vi "QuP Multiplexer Control.vi"(11 "Do full quit? (T)":bool=TRUE) -> ()   [LabVIEW 2020, in "QuPMXdriver.lvlib"]
uses:
  QuPMXdriver.lvlib
  91754cce-ab52-4237-b78a-64c01c446f44.vi
  32ad12f4-2c8c-4504-800a-0d774754ae80.vi
  bf4f7028-8ca7-4759-aadb-7144e2be3c91.vi
  040f1b57-66c1-4072-aa26-6ea72dd8171f.vi
  6aed5eb3-691d-4dc6-b830-00691c629857.vi
  Sequence Editor.vi
  <vilib>/Comparison/Equal/Equal Functor/Equal Functor.lvclass
panel:
  in  "Init-reset":bool caption="Reset after connect:"
  in  "Init-idquery":bool=TRUE caption="ID query after connect:"
  out "FPdisAcon":refnum<vi>[](array[refnum])
  in  "Startup delay (ms)":u32=2000
  in  "disconnect":bool
  out "dummy for event \"check channels\"":bool
  in  "Set to sequence line:":i32=2 min=1 step=1
  in  "set sq line":bool
  out "Connected\nboards":bool[](array[boolean])
  in  "Get sq from MX":bool
  in  "Load sq to MX":bool
  in  "no sequences get":bool
  out "Number of sequence lines:":i32 min=0 step=1
  in  "sequence editor":bool
  out "Guards ref array":refnum<vi>[][](array[refnum])
  in  "G5C1":bool
  in  "G5C2":bool
  in  "G6C1":bool
  in  "G6C2":bool
  in  "G4C1":bool
  in  "G4C2":bool
  in  "G3C1":bool
  in  "G3C2":bool
  in  "G2C1":bool
  in  "G2C2":bool
  in  "G1C1":bool
  in  "G1C2":bool
  out "No. of connected slave boards:":u32
  out "Slaves ref array":refnum<vi>[][](array[refnum])
  in  "S5C1":bool
  in  "S5C2":bool
  in  "S6C1":bool
  in  "S6C2":bool
  in  "S4C1":bool
  in  "S4C2":bool
  in  "S3C1":bool
  in  "S3C2":bool
  in  "S2C1":bool
  in  "S2C2":bool
  in  "S1C1":bool
  in  "S1C2":bool
  in  "connect":bool
  in  "Get Status":bool
  out "Ready?":bool=TRUE
  out "Enabled":bool=TRUE
  in  "check channels":bool
  in  "delay get":bool
  in  "delay set":bool
  in  "Enable\nDelay (ms)":dbl=2.0 min=0.8
  in  "timer get":bool
  in  "timer set":bool
  in  "Timer (ms)":i32=1000 min=0 step=1
  in  "Trigger polarity":enum32{"Positive", "Negative"}(radio)
  in  "Trigger source":enum32{"Internal", "External"}(radio)
  out "FPenAcon":refnum<vi>[](array[refnum])
  in  "Operation":enum32{"Remote", "Local"}(radio)=enum."Local"
  out "ID:":string
  in  "reset":bool
  in  "clear":bool
  in  "stop":bool
  in  "start":bool
  in  "resume":bool
  in  "pause":bool
  in  "Close":bool
  out "error":errorcluster
  in  "VISA":refnum<visa-resource-name>
  # "Connect"
  # "Status"
  # "Channels"
  # "Properties"
  # "Slave boards"
  # "1       2      3      4      5      6"
  # "Channel 1"
  # "Channel 2"
  # "1       2      3      4      5      6"
  # "Guards"
  # "Channel 1"
  # "These are buttons,\nclick it!"
  # "Channel 2"
  # "Sequence"
  # "Error"
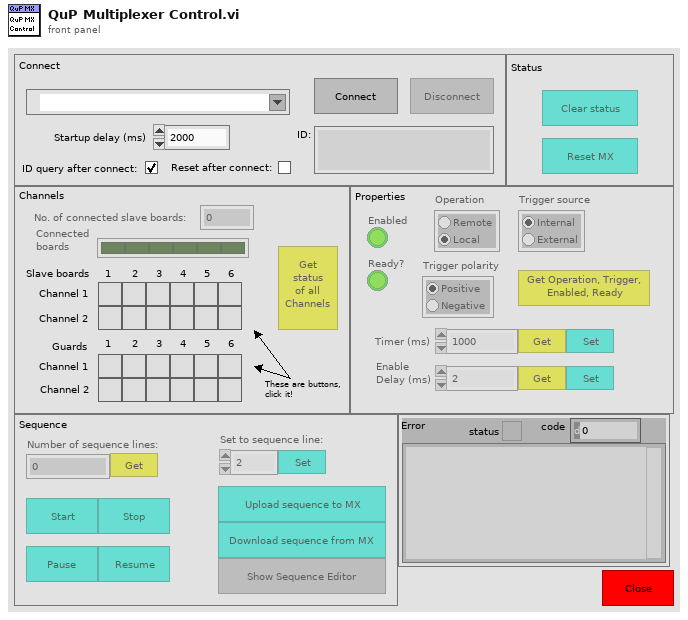
[diagram p1: front panel]
types:
  T1 = enum8{"Enabled", "Disabled", "Disabled and Grayed Out"}
  T2 = enum32{"Invalid", "Standard", "Closed", "Hidden", "Minimized", "Maximized"}
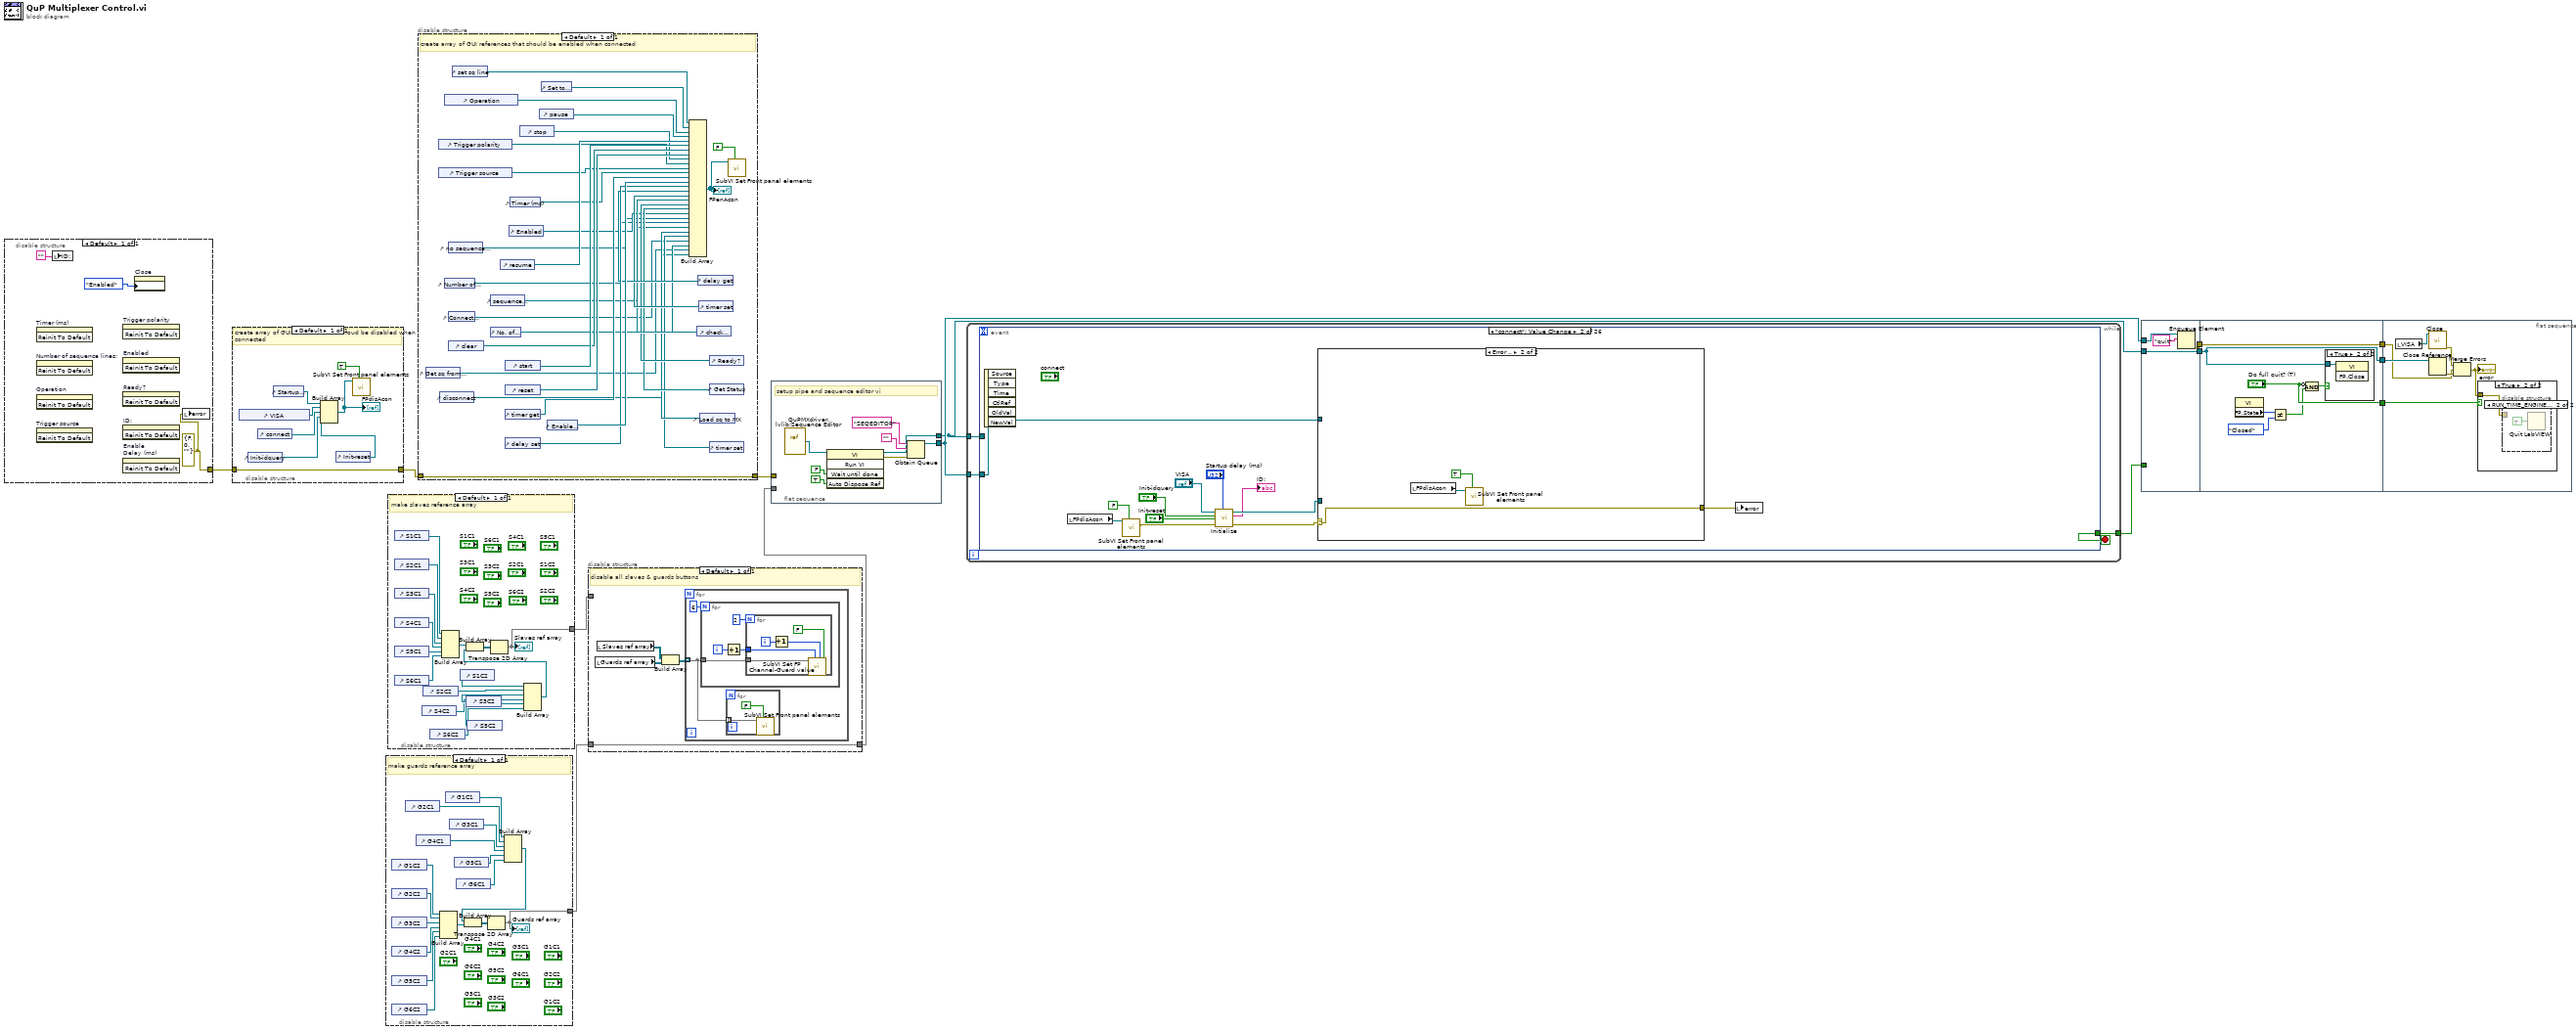
[diagram p0: block diagram]
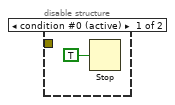
[diagram p4: hidden frame]
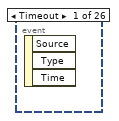
[diagram p5: hidden frame]
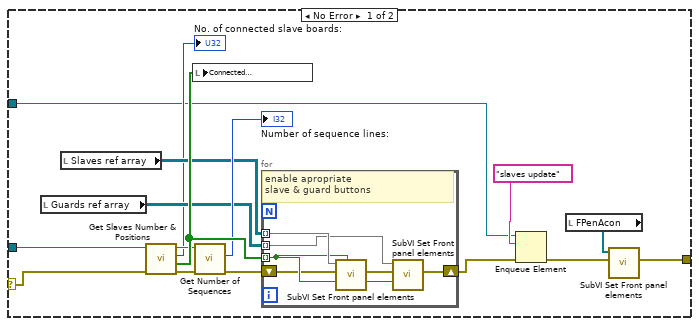
[diagram p6: hidden frame]
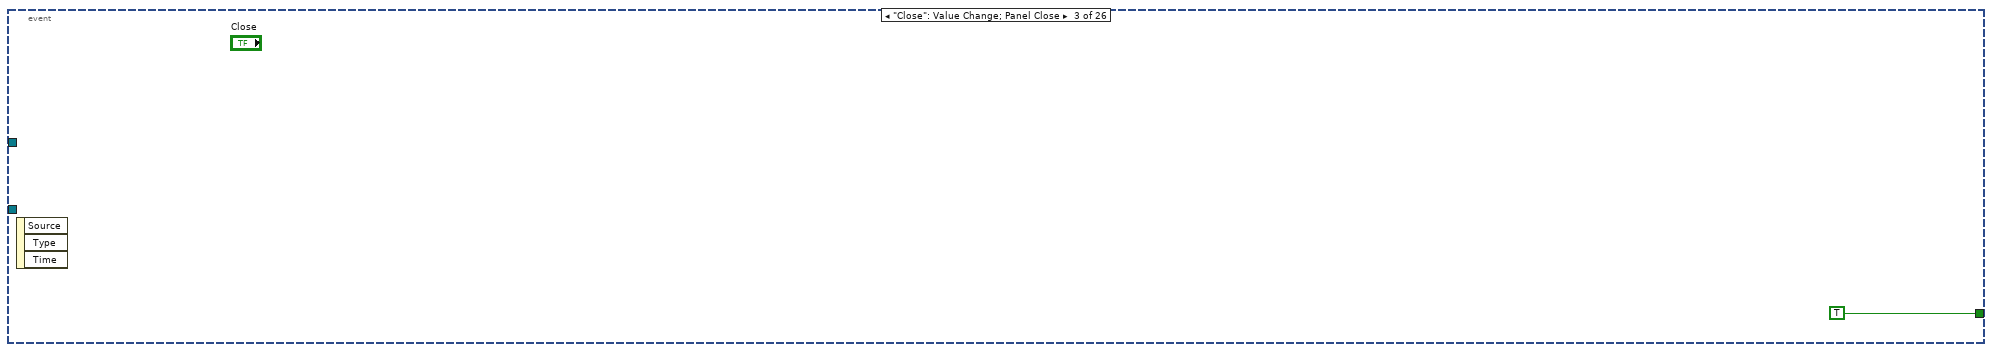
[diagram p7: hidden frame]
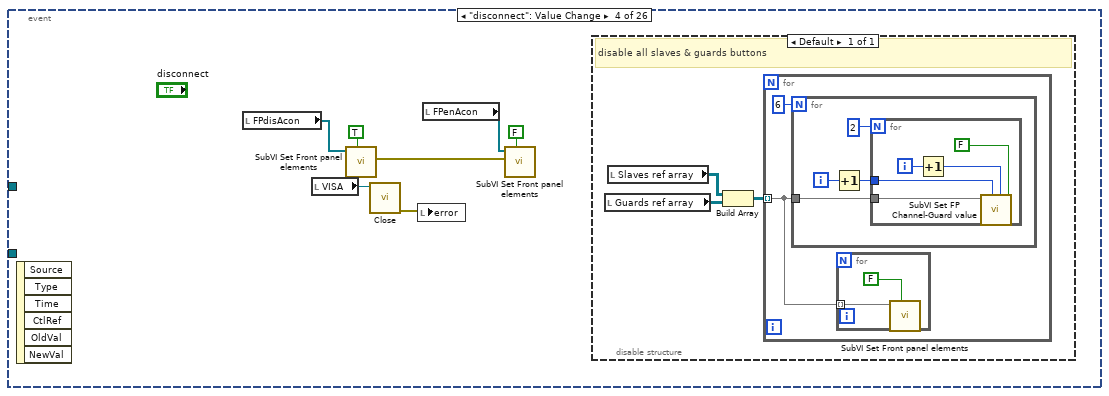
[diagram p8: hidden frame]
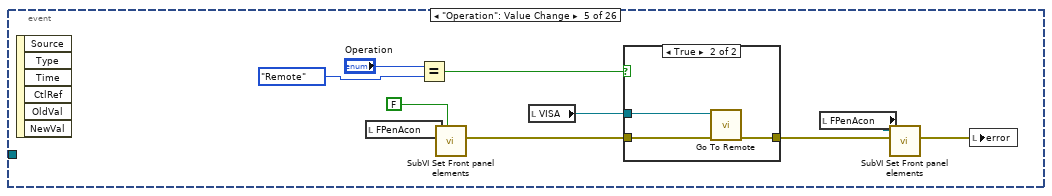
[diagram p9: hidden frame]
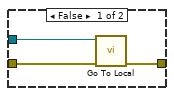
[diagram p10: hidden frame]
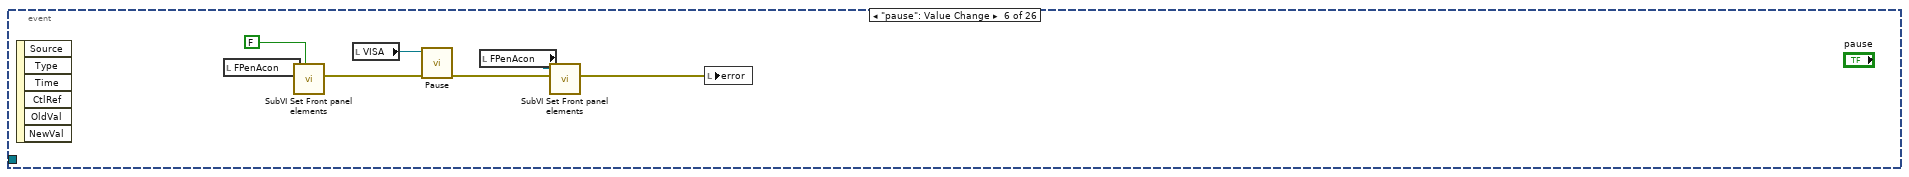
[diagram p11: hidden frame]
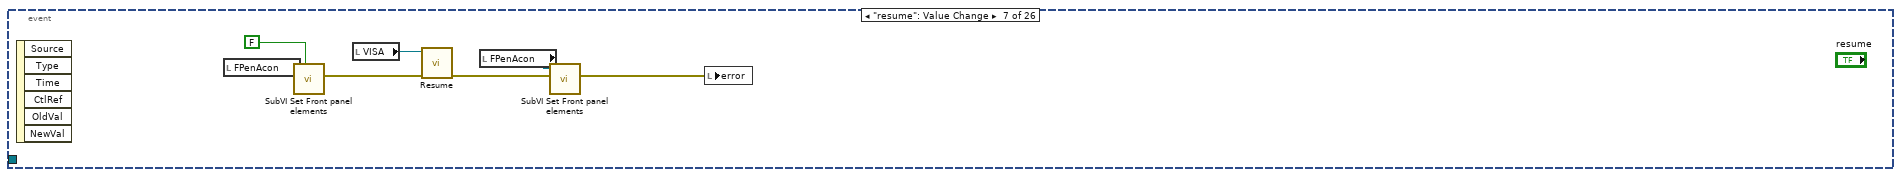
[diagram p12: hidden frame]
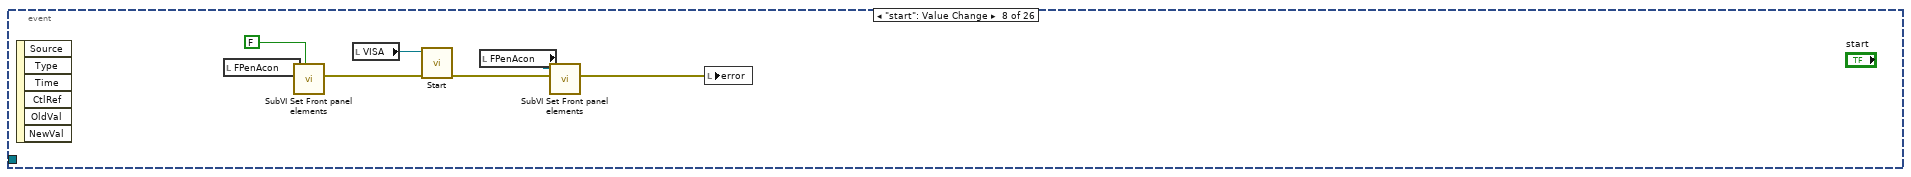
[diagram p13: hidden frame]
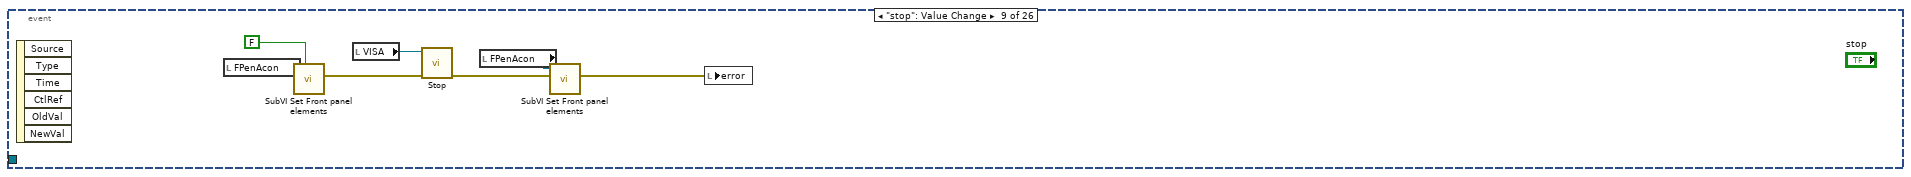
[diagram p14: hidden frame]
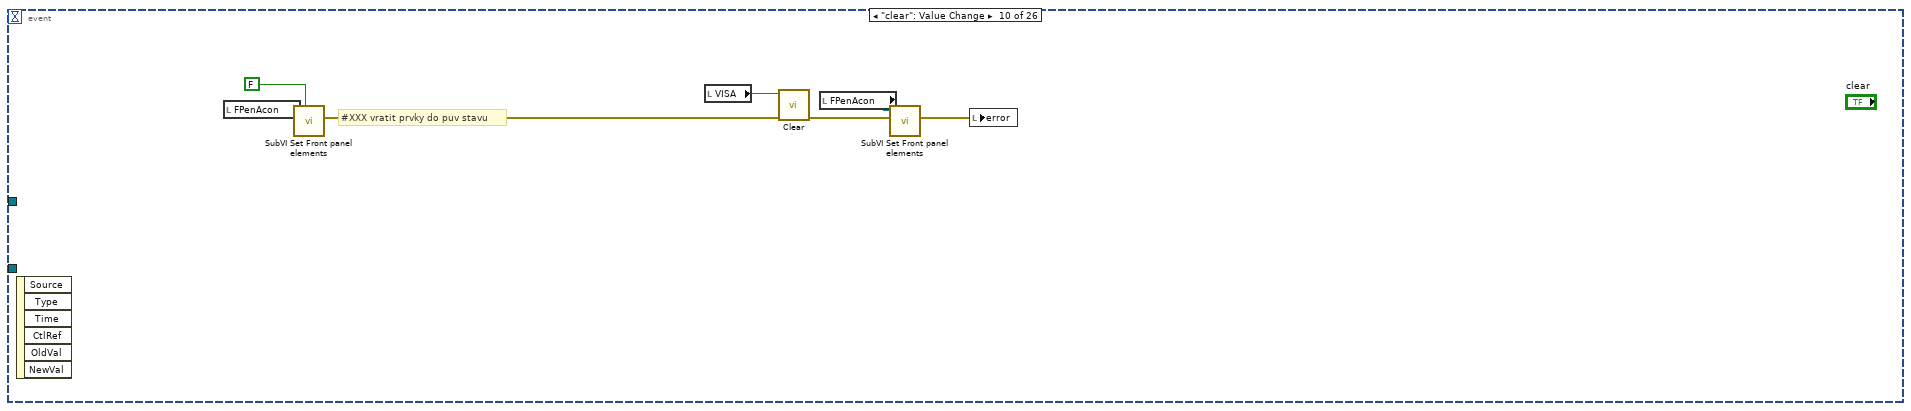
[diagram p15: hidden frame]
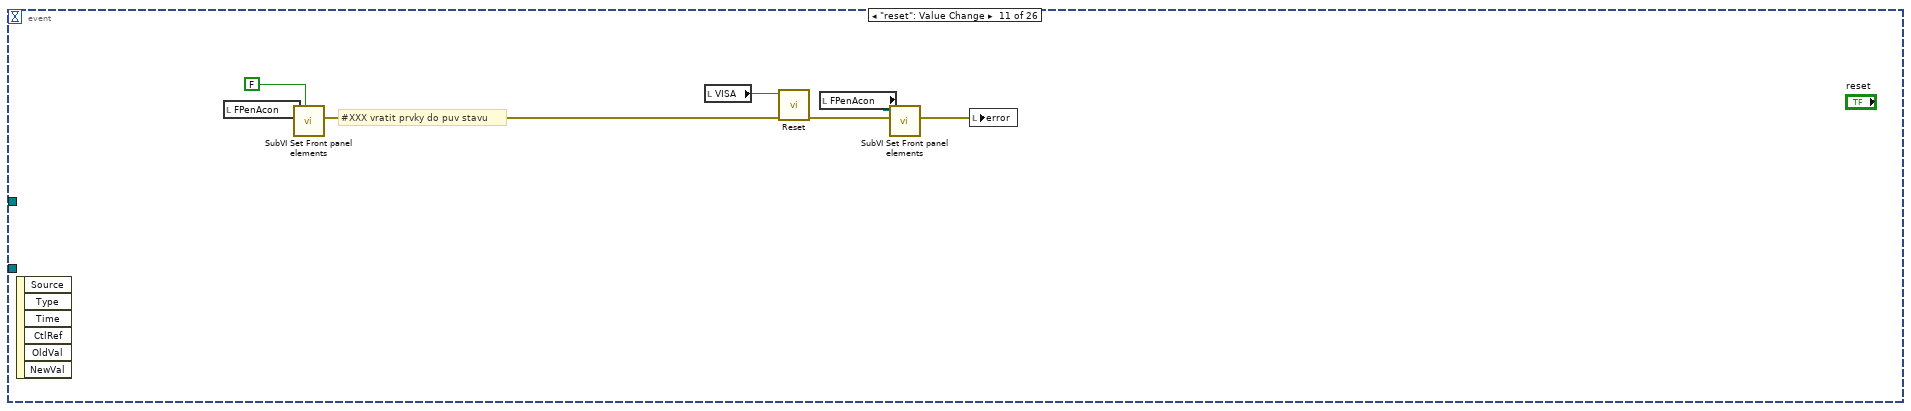
[diagram p16: hidden frame]
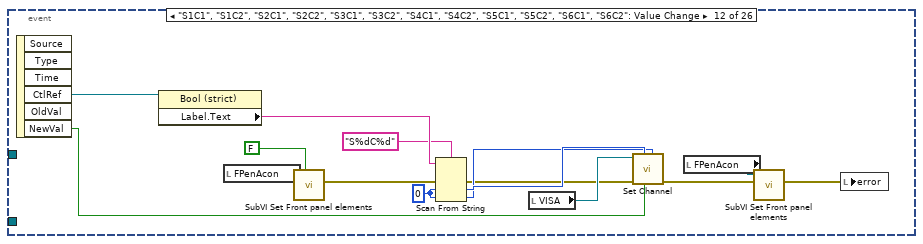
[diagram p17: hidden frame]
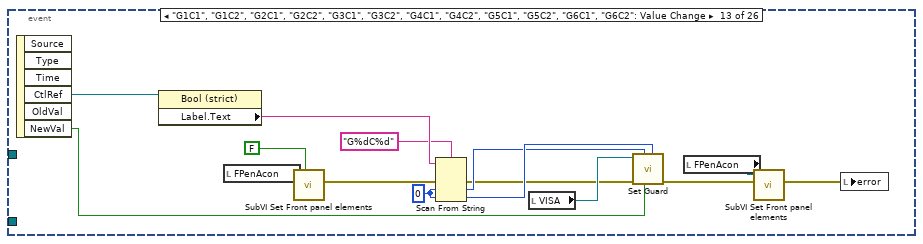
[diagram p18: hidden frame]
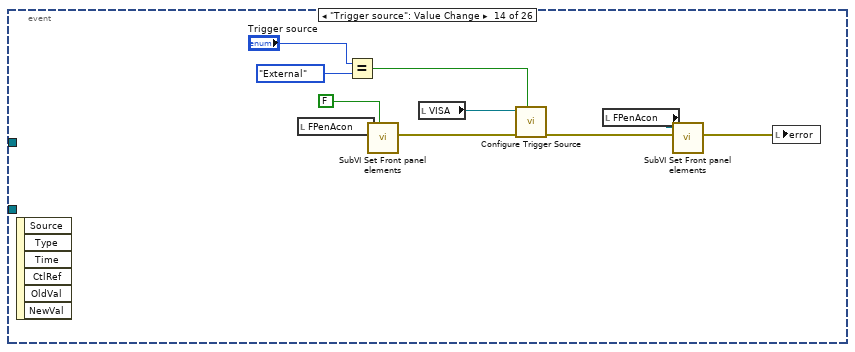
[diagram p19: hidden frame]
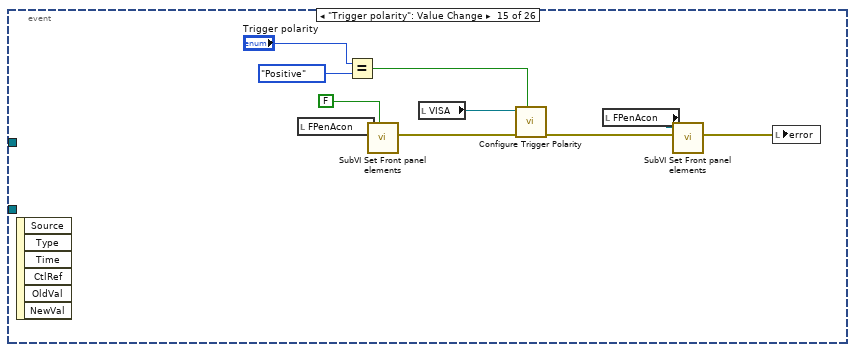
[diagram p20: hidden frame]
diagram:
  n1 = disable-structure shown="Default" {
    disable-tunnel: [w15] -> w1
    frame Enabled {
      w15 = errorcluster {"status"=FALSE, "code"=0, "source"=""} ("error in (no error)")
      n2 = invoke on="Timer (ms)" class="DigNum (strict)" method="Reinit To Default"() -> ()  [unwired: 3 in, 3 out]
      n3 = invoke on="Number of sequence lines:" class="DigNum (strict)" method="Reinit To Default"() -> ()  [unwired: 3 in, 3 out]
      n4 = invoke on="Operation" class="RadioBtnsControl (strict)" method="Reinit To Default"() -> ()  [unwired: 3 in, 3 out]
      n5 = invoke on="Trigger source" class="RadioBtnsControl (strict)" method="Reinit To Default"() -> ()  [unwired: 3 in, 3 out]
      n6 = local write "ID:"("") -> ()
      n7 = invoke on="Trigger polarity" class="RadioBtnsControl (strict)" method="Reinit To Default"() -> ()  [unwired: 3 in, 3 out]
      n8 = invoke on="Enabled" class="Bool (strict)" method="Reinit To Default"() -> ()  [unwired: 3 in, 3 out]
      n9 = invoke on="Ready?" class="Bool (strict)" method="Reinit To Default"() -> ()  [unwired: 3 in, 3 out]
      n10 = invoke on="ID:" class="Str" method="Reinit To Default"() -> ()  [unwired: 3 in, 3 out]
      n11 = invoke on="Enable\nDelay (ms)" class="DigNum (strict)" method="Reinit To Default"() -> ()  [unwired: 3 in, 3 out]
      n12 = property on="Close" class="Bool"("DisabledEnum"=T1."Enabled" ("Disabled")) -> ()  [unwired: 2 in, 2 out]
      n13 = local write "error"(w15) -> ()
    }
  }
  n14 = disable-structure shown="Default" {
    disable-tunnel: [w20] -> w2
    disable-tunnel: w1 -> [w20]
    frame Enabled {
      # "create array of GUI references that shoud be disabled when connected"
      n15 = control-ref of="VISA"() -> (w24:refnum<vi>)
      n16 = control-ref of="Init-idquery"() -> (w19:refnum<vi>)
      n17 = control-ref of="connect"() -> (w23:refnum<vi>)
      n18 = control-ref of="Startup delay (ms)"() -> (w25:refnum<vi>)
      n19 = control-ref of="Init-reset"() -> (w18:refnum<vi>)
      n20 = Build Array(w25, w24, w23, w19, w18) -> (w21:refnum<vi>[])
      "FPdisAcon" <- w21
      n21 = call "SubVI Set Front panel elements.vi"("Enable elements (T)"=TRUE ("Enable elements"), "Array"=w21) -> ()  [unwired: 9 in, 1 out]
    }
  }
  n22 = disable-structure shown="Default" {
    disable-tunnel: [w26] -> w12
    frame Enabled {
      # "make guards reference array"
      n23 = control-ref of="G1C2"() -> (w27:refnum<vi>)
      n24 = control-ref of="G2C2"() -> (w28:refnum<vi>)
      n25 = control-ref of="G3C2"() -> (w29:refnum<vi>)
      n26 = control-ref of="G4C2"() -> (w30:refnum<vi>)
      n27 = control-ref of="G5C2"() -> (w31:refnum<vi>)
      n28 = control-ref of="G6C2"() -> (w32:refnum<vi>)
      n29 = control-ref of="G2C1"() -> (w35:refnum<vi>)
      n30 = control-ref of="G4C1"() -> (w37:refnum<vi>)
      n31 = Build Array(w27, w28, w29, w30, w31, w32) -> (w40:refnum<vi>[])
      n32 = control-ref of="G1C1"() -> (w34:refnum<vi>)
      n33 = control-ref of="G3C1"() -> (w36:refnum<vi>)
      n34 = control-ref of="G5C1"() -> (w38:refnum<vi>)
      n35 = control-ref of="G6C1"() -> (w39:refnum<vi>)
      n36 = Build Array(w34, w35, w36, w37, w38, w39) -> (w33:refnum<vi>[])
      n37 = Build Array(w33, w40) -> (w41:refnum<vi>[][])
      n38 = Transpose 2D Array(2D array=w41) -> (transposed array=w26:refnum<vi>[][])
      "Guards ref array" <- w26
    }
  }
  n39 = disable-structure shown="Default" {
    disable-tunnel: [w42] -> w13
    frame Enabled {
      # "make slaves reference array"
      n40 = control-ref of="S1C1"() -> (w57:refnum<vi>)
      n41 = control-ref of="S2C1"() -> (w56:refnum<vi>)
      n42 = control-ref of="S3C1"() -> (w55:refnum<vi>)
      n43 = control-ref of="S4C1"() -> (w54:refnum<vi>)
      n44 = control-ref of="S5C1"() -> (w53:refnum<vi>)
      n45 = control-ref of="S6C1"() -> (w52:refnum<vi>)
      n46 = control-ref of="S4C2"() -> (w48:refnum<vi>)
      n47 = control-ref of="S2C2"() -> (w50:refnum<vi>)
      n48 = control-ref of="S6C2"() -> (w46:refnum<vi>)
      n49 = Build Array(w57, w56, w55, w54, w53, w52) -> (w44:refnum<vi>[])
      n50 = control-ref of="S1C2"() -> (w51:refnum<vi>)
      n51 = control-ref of="S3C2"() -> (w49:refnum<vi>)
      n52 = control-ref of="S5C2"() -> (w47:refnum<vi>)
      n53 = Build Array(w51, w50, w49, w48, w47, w46) -> (w45:refnum<vi>[])
      n54 = Build Array(w44, w45) -> (w43:refnum<vi>[][])
      n55 = Transpose 2D Array(2D array=w43) -> (transposed array=w42:refnum<vi>[][])
      "Slaves ref array" <- w42
    }
  }
  n56 = disable-structure shown="Default" {
    disable-tunnel: [w65] -> w8
    disable-tunnel: w2 -> [w65]
    frame Enabled {
      # "create array of GUI references that should be enabled when connected"
      n57 = control-ref of="Get sq from MX"() -> (w61:refnum<vi>)
      n58 = control-ref of="Trigger polarity"() -> (w81:refnum<vi>)
      n59 = control-ref of="Trigger source"() -> (w80:refnum<vi>)
      n60 = control-ref of="disconnect"() -> (w58:refnum<vi>)
      n61 = control-ref of="Operation"() -> (w90:refnum<vi>)
      n62 = control-ref of="Number of sequence lines:"() -> (w68:refnum<vi>)
      n63 = control-ref of="no sequences get"() -> (w69:refnum<vi>)
      n64 = control-ref of="Connected\nboards"() -> (w63:refnum<vi>)
      n65 = control-ref of="clear"() -> (w86:refnum<vi>)
      n66 = control-ref of="set sq line"() -> (w59:refnum<vi>)
      n67 = control-ref of="sequence editor"() -> (w67:refnum<vi>)
      n68 = control-ref of="No. of connected slave boards:"() -> (w62:refnum<vi>)
      n69 = control-ref of="resume"() -> (w88:refnum<vi>)
      n70 = control-ref of="start"() -> (w87:refnum<vi>)
      n71 = control-ref of="reset"() -> (w85:refnum<vi>)
      n72 = control-ref of="timer get"() -> (w78:refnum<vi>)
      n73 = control-ref of="delay set"() -> (w76:refnum<vi>)
      n74 = control-ref of="Enabled"() -> (w70:refnum<vi>)
      n75 = control-ref of="Timer (ms)"() -> (w79:refnum<vi>)
      n76 = control-ref of="stop"() -> (w82:refnum<vi>)
      n77 = control-ref of="pause"() -> (w89:refnum<vi>)
      n78 = control-ref of="Set to sequence line:"() -> (w60:refnum<vi>)
      n79 = control-ref of="Enable\nDelay (ms)"() -> (w77:refnum<vi>)
      n80 = control-ref of="check channels"() -> (w73:refnum<vi>)
      n81 = control-ref of="delay get"() -> (w75:refnum<vi>)
      n82 = control-ref of="timer set"() -> (w74:refnum<vi>)
      n83 = control-ref of="Load sq to MX"() -> (w66:refnum<vi>)
      n84 = control-ref of="Ready?"() -> (w72:refnum<vi>)
      n85 = control-ref of="Get Status"() -> (w71:refnum<vi>)
      n86 = control-ref of="timer set"() -> (w64:refnum<vi>)
      n87 = Build Array(w59, w60, w90, w89, w88, w87, w86, w85, w82, w81, w80, w79, w78, w77, w76, w75, w74, w73, w72, w71, w70, w69, w68, w67, w66, w64, w63, w62, w61, w58) -> (w84:refnum<vi>[])
      "FPenAcon" <- w84
      n88 = call "SubVI Set Front panel elements.vi"("Enable elements (T)"=FALSE ("Enable elements"), "Array"=w84) -> ()  [unwired: 9 in, 1 out]
    }
  }
  n89 = disable-structure shown="Default" {
    disable-tunnel: w13 -> [_]
    disable-tunnel: w12 -> [w91]
    disable-tunnel: [w91] -> w9
    frame Enabled {
      # "disable all slaves & guards buttons"
      n90 = local read "Guards ref array"() -> (w92:refnum<vi>[][])
      n91 = local read "Slaves ref array"() -> (w94:refnum<vi>[][])
      n92 = Build Array(w94, w92) -> (w93:refnum<vi>[][][])
      n93 = for {
        tunnel: w93 -> [w95] mode=indexing
        n94 = for {
          N: 6 -> [_]
          tunnel: w95 -> [w100]
          i -> [w98]
          n95 = Increment(x=w98) -> (x+1=w97:i32)
          n96 = for {
            N: 2 -> [_]
            tunnel: w100 -> [w105]
            tunnel: w97 -> [w103]
            i -> [w102]
            n97 = Increment(x=w102) -> (x+1=w101:i32)
            n98 = call "SubVI Set FP Channel-Guard value.vi"("Value"=FALSE, "Ch ID"=w101, "Slave ID"=w103, "Slaves ref array"=w105) -> ()  [unwired: 7 in, 1 out]
          }
        }
        n99 = for {
          tunnel: w95 -> [w107] mode=indexing
          n100 = call "SubVI Set Front panel elements.vi"("Enable elements (T)"=FALSE, "Array"=w107) -> ()  [unwired: 9 in, 1 out]
        }
      }
    }
  }
  n101 = flat-sequence {
    tunnel: [w108] -> w11
    tunnel: [w110] -> w10
    tunnel: w9 -> [_]
    tunnel: w8 -> [_]
    frame #0 {
      # "setup pipe and sequence editor vi"
      n102 = vi-ref "QuPMXdriver.lvlib:Sequence Editor.vi"() -> (w115:refnum<vi>)
      n103 = invoke class="VI" method="Run VI"(reference=w115, "Wait until done"=FALSE ("Wait Until Done"), "Auto Dispose Ref"=TRUE ("Wait Until Done")) -> (reference out=w110:refnum<vi>, error out=w111:errorcluster)  [unwired: 2 in, 3 out]
      n104 = Obtain Queue(name (unnamed)="SEQEDITOR", element data type="", error in (no error)=w111) -> (queue out=w108:refnum<queue>)  [unwired: 2 in, 2 out]
    }
  }
  n105 = while {
    tunnel: [w118] -> w14
    tunnel: w11 -> [w117]
    tunnel: w10 -> [w116]
    stop <- w118 stop-if-true
    n106 = event shown="[1] \"connect\": Value Change" {
      selector: _ -> [_ _ _ _ _ _ _ _ _ _ _ _ _ _ _ _ _ _ _ _ _ _ _ _ _ _]
      dyn-events: _ -> [_ _ _ _ _ _ _ _ _ _ _ _ _ _ _ _ _ _ _ _ _ _ _ _ _ _]
      timeout: _ -> [_ _ _ _ _ _ _ _ _ _ _ _ _ _ _ _ _ _ _ _ _ _ _ _ _ _]
      tunnel: [_ _ TRUE ("Stop") _ _ _ _ _ _ _ _ _ _ _ _ _ _ _ _ _ _ _ _ _ _ _] -> w118
      tunnel: w117 -> [_ w127 _ _ _ _ _ _ _ _ _ _ _ _ _ _ _ _ _ w327 _ _ w391 _ _ w468]
      tunnel: w116 -> [_ _ _ _ _ _ _ _ _ _ _ _ _ _ _ _ _ _ _ _ _ _ _ w396 w444 w471]
      event Timeout {
        n107 = event-data() -> ()  [unwired: 1 in, 3 out]
      }
      event "connect": Value Change {
        n108 = event-data() -> ()  [unwired: 1 in, 6 out]
        n109 = local read "FPdisAcon"() -> (w124:refnum<vi>[])
        n110 = call "SubVI Set Front panel elements.vi"("Enable elements (T)"=FALSE, "Array"=w124) -> ("error out"=w122:errorcluster)  [unwired: 9 in]
        n111 = call "Initialize.vi"("Startup delay (0 ms)"="Startup delay (ms)", "error in (no error)"=w122, "Reset (False)"="Init-reset", "ID Query (True)"="Init-idquery", "VISA resource name"="VISA") -> ("error out"=w121:errorcluster, "ID"=→"ID:":string, "VISA resource name out"=w129:refnum<visa-resource-name>)  [unwired: 4 in]
        n112 = case shown="Error .." w121 {
          selector: w121 -> [w131 w155]
          tunnel: w129 -> [w138 _]
          tunnel: w127 -> [w133 _]
          tunnel: [w132 w155] -> w125
          frame No Error {
            n113 = local read "Guards ref array"() -> (w141:refnum<vi>[][])
            n114 = local read "Slaves ref array"() -> (w140:refnum<vi>[][])
            n115 = call "Get Slaves Number & Positions.vi"("error in (no error)"=w131, "VISA resource name"=w138) -> ("error out"=w142:errorcluster, "Connected Slaves"=w146:bool[], "No. of Slaves"=→"No. of connected slave boards:":u32, "VISA resource name out"=w144:refnum<visa-resource-name>)  [unwired: 6 in]
            n116 = local write "Connected\nboards"(w146) -> ()
            n117 = call "Get Number of Sequences.vi"("error in (no error)"=w142, "VISA resource name"=w144) -> ("error out"=w143:errorcluster, "Number of sequences"=→"Number of sequence lines:":i32)  [unwired: 7 in, 1 out]
            n118 = for {
              tunnel: w140 -> [w152] mode=indexing
              tunnel: w146 -> [w150] mode=indexing
              tunnel: w141 -> [w151] mode=indexing
              shift-right: [w148] -> w134
              shift-left: w143 -> [w147]
              # "enable apropriate\nslave & guard buttons"
              n119 = call "SubVI Set Front panel elements.vi"("Enable elements (T)"=w150, "error in (passthrough)"=w147, "Array"=w152) -> ("error out"=w149:errorcluster)  [unwired: 8 in]
              n120 = call "SubVI Set Front panel elements.vi"("Enable elements (T)"=w150, "error in (passthrough)"=w149, "Array"=w151) -> ("error out"=w148:errorcluster)  [unwired: 8 in]
            }
            n121 = Enqueue Element(queue=w133, element="slaves update", error in (no error)=w134) -> (error out=w137:errorcluster)  [unwired: 1 in, 2 out]
            n122 = local read "FPenAcon"() -> (w136:refnum<vi>[])
            n123 = call "SubVI Set Front panel elements.vi"("error in (passthrough)"=w137, "Array"=w136) -> ("error out"=w132:errorcluster)  [unwired: 9 in]
          }
          frame Error {
            n124 = local read "FPdisAcon"() -> (w153:refnum<vi>[])
            n125 = call "SubVI Set Front panel elements.vi"("Enable elements (T)"=TRUE, "Array"=w153) -> ()  [unwired: 9 in, 1 out]
          }
        }
        n126 = local write "error"(w125) -> ()
      }
      event "Close": Value Change; Panel Close {
        n127 = event-data() -> ()  [unwired: 1 in, 3 out]
      }
      event "disconnect": Value Change {
        n128 = event-data() -> ()  [unwired: 1 in, 6 out]
        n129 = local read "FPdisAcon"() -> (w158:refnum<vi>[])
        n130 = local read "VISA"() -> (w163:refnum<visa-resource-name>)
        n131 = call "SubVI Set Front panel elements.vi"("Enable elements (T)"=TRUE, "Array"=w158) -> ("error out"=w159:errorcluster)  [unwired: 9 in]
        n132 = call "Close.vi"("VISA resource name"=w163) -> ("error out"=w162:errorcluster)  [unwired: 10 in]
        n133 = local write "error"(w162) -> ()
        n134 = local read "FPenAcon"() -> (w161:refnum<vi>[])
        n135 = call "SubVI Set Front panel elements.vi"("Enable elements (T)"=FALSE, "error in (passthrough)"=w159, "Array"=w161) -> ()  [unwired: 8 in, 1 out]
        n136 = disable-structure shown="Default" {
          frame Enabled {
            # "disable all slaves & guards buttons"
            n137 = local read "Guards ref array"() -> (w164:refnum<vi>[][])
            n138 = local read "Slaves ref array"() -> (w166:refnum<vi>[][])
            n139 = Build Array(w166, w164) -> (w165:refnum<vi>[][][])
            n140 = for {
              tunnel: w165 -> [w167] mode=indexing
              n141 = for {
                N: 6 -> [_]
                tunnel: w167 -> [w172]
                i -> [w170]
                n142 = Increment(x=w170) -> (x+1=w169:i32)
                n143 = for {
                  N: 2 -> [_]
                  tunnel: w172 -> [w177]
                  tunnel: w169 -> [w175]
                  i -> [w174]
                  n144 = Increment(x=w174) -> (x+1=w173:i32)
                  n145 = call "SubVI Set FP Channel-Guard value.vi"("Value"=FALSE, "Ch ID"=w173, "Slave ID"=w175, "Slaves ref array"=w177) -> ()  [unwired: 7 in, 1 out]
                }
              }
              n146 = for {
                tunnel: w167 -> [w179] mode=indexing
                n147 = call "SubVI Set Front panel elements.vi"("Enable elements (T)"=FALSE, "Array"=w179) -> ()  [unwired: 9 in, 1 out]
              }
            }
          }
        }
      }
      event "Operation": Value Change {
        n148 = event-data() -> ()  [unwired: 1 in, 6 out]
        n149 = local read "FPenAcon"() -> (w185:refnum<vi>[])
        n150 = Equal?(x="Operation", y=enum32{"Remote", "Local"}."Remote") -> (x = y?=w186:bool)
        n151 = call "SubVI Set Front panel elements.vi"("Enable elements (T)"=FALSE, "Array"=w185) -> ("error out"=w183:errorcluster)  [unwired: 9 in]
        n152 = local read "VISA"() -> (w189:refnum<visa-resource-name>)
        n153 = case shown="True" w186 {
          tunnel: [w192 w195] -> w182
          tunnel: w189 -> [w191 w194]
          tunnel: w183 -> [w190 w193]
          frame False {
            n154 = call "Go To Local.vi"("error in (no error)"=w190, "VISA resource name"=w191) -> ("error out"=w192:errorcluster)  [unwired: 8 in, 1 out]
          }
          frame True {
            n155 = call "Go To Remote.vi"("error in (no error)"=w193, "VISA resource name"=w194) -> ("error out"=w195:errorcluster)  [unwired: 8 in, 1 out]
          }
        }
        n156 = local read "FPenAcon"() -> (w180:refnum<vi>[])
        n157 = call "SubVI Set Front panel elements.vi"("error in (passthrough)"=w182, "Array"=w180) -> ("error out"=w181:errorcluster)  [unwired: 9 in]
        n158 = local write "error"(w181) -> ()
      }
      event "pause": Value Change {
        n159 = event-data() -> ()  [unwired: 1 in, 6 out]
        n160 = local read "FPenAcon"() -> (w201:refnum<vi>[])
        n161 = call "SubVI Set Front panel elements.vi"("Enable elements (T)"=FALSE, "Array"=w201) -> ("error out"=w198:errorcluster)  [unwired: 9 in]
        n162 = local read "VISA"() -> (w202:refnum<visa-resource-name>)
        n163 = call "Pause.vi"("error in (no error)"=w198, "VISA resource name"=w202) -> ("error out"=w197:errorcluster)  [unwired: 8 in, 1 out]
        n164 = local read "FPenAcon"() -> (w199:refnum<vi>[])
        n165 = call "SubVI Set Front panel elements.vi"("error in (passthrough)"=w197, "Array"=w199) -> ("error out"=w196:errorcluster)  [unwired: 9 in]
        n166 = local write "error"(w196) -> ()
      }
      event "resume": Value Change {
        n167 = event-data() -> ()  [unwired: 1 in, 6 out]
        n168 = local read "FPenAcon"() -> (w207:refnum<vi>[])
        n169 = call "SubVI Set Front panel elements.vi"("Enable elements (T)"=FALSE, "Array"=w207) -> ("error out"=w205:errorcluster)  [unwired: 9 in]
        n170 = local read "VISA"() -> (w209:refnum<visa-resource-name>)
        n171 = call "Resume.vi"("error in (no error)"=w205, "VISA resource name"=w209) -> ("error out"=w204:errorcluster)  [unwired: 8 in, 1 out]
        n172 = local read "FPenAcon"() -> (w208:refnum<vi>[])
        n173 = call "SubVI Set Front panel elements.vi"("error in (passthrough)"=w204, "Array"=w208) -> ("error out"=w203:errorcluster)  [unwired: 9 in]
        n174 = local write "error"(w203) -> ()
      }
      event "start": Value Change {
        n175 = event-data() -> ()  [unwired: 1 in, 6 out]
        n176 = local read "FPenAcon"() -> (w214:refnum<vi>[])
        n177 = call "SubVI Set Front panel elements.vi"("Enable elements (T)"=FALSE, "Array"=w214) -> ("error out"=w212:errorcluster)  [unwired: 9 in]
        n178 = local read "VISA"() -> (w216:refnum<visa-resource-name>)
        n179 = call "Start.vi"("error in (no error)"=w212, "VISA resource name"=w216) -> ("error out"=w211:errorcluster)  [unwired: 8 in, 1 out]
        n180 = local read "FPenAcon"() -> (w215:refnum<vi>[])
        n181 = call "SubVI Set Front panel elements.vi"("error in (passthrough)"=w211, "Array"=w215) -> ("error out"=w210:errorcluster)  [unwired: 9 in]
        n182 = local write "error"(w210) -> ()
      }
      event "stop": Value Change {
        n183 = event-data() -> ()  [unwired: 1 in, 6 out]
        n184 = local read "FPenAcon"() -> (w221:refnum<vi>[])
        n185 = call "SubVI Set Front panel elements.vi"("Enable elements (T)"=FALSE, "Array"=w221) -> ("error out"=w219:errorcluster)  [unwired: 9 in]
        n186 = local read "VISA"() -> (w223:refnum<visa-resource-name>)
        n187 = call "Stop.vi"("error in (no error)"=w219, "VISA resource name"=w223) -> ("error out"=w218:errorcluster)  [unwired: 8 in, 1 out]
        n188 = local read "FPenAcon"() -> (w222:refnum<vi>[])
        n189 = call "SubVI Set Front panel elements.vi"("error in (passthrough)"=w218, "Array"=w222) -> ("error out"=w217:errorcluster)  [unwired: 9 in]
        n190 = local write "error"(w217) -> ()
      }
      event "clear": Value Change {
        # "#XXX vratit prvky do puv stavu"
        n191 = event-data() -> ()  [unwired: 1 in, 6 out]
        n192 = local read "FPenAcon"() -> (w228:refnum<vi>[])
        n193 = call "SubVI Set Front panel elements.vi"("Enable elements (T)"=FALSE, "Array"=w228) -> ("error out"=w226:errorcluster)  [unwired: 9 in]
        n194 = local read "VISA"() -> (w230:refnum<visa-resource-name>)
        n195 = call "Clear.vi"("error in (no error)"=w226, "VISA resource name"=w230) -> ("error out"=w225:errorcluster)  [unwired: 8 in, 1 out]
        n196 = local read "FPenAcon"() -> (w229:refnum<vi>[])
        n197 = call "SubVI Set Front panel elements.vi"("error in (passthrough)"=w225, "Array"=w229) -> ("error out"=w224:errorcluster)  [unwired: 9 in]
        n198 = local write "error"(w224) -> ()
      }
      event "reset": Value Change {
        # "#XXX vratit prvky do puv stavu"
        n199 = event-data() -> ()  [unwired: 1 in, 6 out]
        n200 = local read "FPenAcon"() -> (w235:refnum<vi>[])
        n201 = call "SubVI Set Front panel elements.vi"("Enable elements (T)"=FALSE, "Array"=w235) -> ("error out"=w233:errorcluster)  [unwired: 9 in]
        n202 = local read "VISA"() -> (w237:refnum<visa-resource-name>)
        n203 = call "Reset.vi"("error in (no error)"=w233, "VISA resource name"=w237) -> ("error out"=w232:errorcluster)  [unwired: 8 in, 1 out]
        n204 = local read "FPenAcon"() -> (w236:refnum<vi>[])
        n205 = call "SubVI Set Front panel elements.vi"("error in (passthrough)"=w232, "Array"=w236) -> ("error out"=w231:errorcluster)  [unwired: 9 in]
        n206 = local write "error"(w231) -> ()
      }
      event "S1C1", "S1C2", "S2C1", "S2C2", "S3C1", "S3C2", "S4C1", "S4C2", "S5C1", "S5C2", "S6C1", "S6C2": Value Change {
        w238 = 0 ("default value 1")
        n207 = event-data() -> ("CtlRef"=w252:refnum<vi>, "NewVal"=w246:bool)  [unwired: 1 in, 4 out]
        n208 = property class="Bool (strict)"(reference=w252) -> ("Label.Text"=w251:string)  [unwired: 1 in, 2 out]
        n209 = local read "FPenAcon"() -> (w241:refnum<vi>[])
        n210 = call "SubVI Set Front panel elements.vi"("Enable elements (T)"=FALSE, "Array"=w241) -> ("error out"=w239:errorcluster)  [unwired: 9 in]
        n211 = Scan From String(format string="S%dC%d", input string=w251, error in=w239, default 1=w238, default 2=w238) -> (error out=w245:errorcluster, output 1=w249:i32, output 2=w248:i32)  [unwired: 1 in, 2 out]
        n212 = local read "VISA"() -> (w247:refnum<visa-resource-name>)
        n213 = call "Set Channel.vi"("Channel"=w248, "Channel Status"=w246, "Slave"=w249, "error in (no error)"=w245, "VISA resource name"=w247) -> ("error out"=w243:errorcluster)  [unwired: 5 in, 1 out]
        n214 = local read "FPenAcon"() -> (w244:refnum<vi>[])
        n215 = call "SubVI Set Front panel elements.vi"("error in (passthrough)"=w243, "Array"=w244) -> ("error out"=w242:errorcluster)  [unwired: 9 in]
        n216 = local write "error"(w242) -> ()
      }
      event "G1C1", "G1C2", "G2C1", "G2C2", "G3C1", "G3C2", "G4C1", "G4C2", "G5C1", "G5C2", "G6C1", "G6C2": Value Change {
        w259 = 0 ("default value 1")
        n217 = event-data() -> ("CtlRef"=w265:refnum<vi>, "NewVal"=w261:bool)  [unwired: 1 in, 4 out]
        n218 = property class="Bool (strict)"(reference=w265) -> ("Label.Text"=w267:string)  [unwired: 1 in, 2 out]
        n219 = local read "FPenAcon"() -> (w258:refnum<vi>[])
        n220 = call "SubVI Set Front panel elements.vi"("Enable elements (T)"=FALSE, "Array"=w258) -> ("error out"=w256:errorcluster)  [unwired: 9 in]
        n221 = Scan From String(format string="G%dC%d", input string=w267, error in=w256, default 1=w259, default 2=w259) -> (error out=w260:errorcluster, output 1=w263:i32, output 2=w264:i32)  [unwired: 1 in, 2 out]
        n222 = local read "VISA"() -> (w262:refnum<visa-resource-name>)
        n223 = call "Set Guard.vi"("Channel"=w264, "Channel Guard Status"=w261, "Slave"=w263, "error in (no error)"=w260, "VISA resource name"=w262) -> ("error out"=w254:errorcluster)  [unwired: 5 in, 1 out]
        n224 = local read "FPenAcon"() -> (w255:refnum<vi>[])
        n225 = call "SubVI Set Front panel elements.vi"("error in (passthrough)"=w254, "Array"=w255) -> ("error out"=w253:errorcluster)  [unwired: 9 in]
        n226 = local write "error"(w253) -> ()
      }
      event "Trigger source": Value Change {
        n227 = event-data() -> ()  [unwired: 1 in, 6 out]
        n228 = local read "FPenAcon"() -> (w275:refnum<vi>[])
        n229 = Equal?(x="Trigger source", y=enum32{"Internal", "External"}."External") -> (x = y?=w269:bool)
        n230 = call "SubVI Set Front panel elements.vi"("Enable elements (T)"=FALSE, "Array"=w275) -> ("error out"=w271:errorcluster)  [unwired: 9 in]
        n231 = local read "VISA"() -> (w273:refnum<visa-resource-name>)
        n232 = call "Configure Trigger Source.vi"("Trigger External (T)"=w269, "error in (no error)"=w271, "VISA resource name"=w273) -> ("error out"=w272:errorcluster)  [unwired: 7 in, 1 out]
        n233 = local read "FPenAcon"() -> (w276:refnum<vi>[])
        n234 = call "SubVI Set Front panel elements.vi"("error in (passthrough)"=w272, "Array"=w276) -> ("error out"=w277:errorcluster)  [unwired: 9 in]
        n235 = local write "error"(w277) -> ()
      }
      event "Trigger polarity": Value Change {
        n236 = event-data() -> ()  [unwired: 1 in, 6 out]
        n237 = local read "FPenAcon"() -> (w285:refnum<vi>[])
        n238 = Equal?(x="Trigger polarity", y=enum32{"Positive", "Negative"}."Positive") -> (x = y?=w279:bool)
        n239 = call "SubVI Set Front panel elements.vi"("Enable elements (T)"=FALSE, "Array"=w285) -> ("error out"=w283:errorcluster)  [unwired: 9 in]
        n240 = local read "VISA"() -> (w278:refnum<visa-resource-name>)
        n241 = call "Configure Trigger Polarity.vi"("Trigger Polarity Positive (T)"=w279, "error in (no error)"=w283, "VISA resource name"=w278) -> ("error out"=w282:errorcluster)  [unwired: 7 in, 1 out]
        n242 = local read "FPenAcon"() -> (w286:refnum<vi>[])
        n243 = call "SubVI Set Front panel elements.vi"("error in (passthrough)"=w282, "Array"=w286) -> ("error out"=w287:errorcluster)  [unwired: 9 in]
        n244 = local write "error"(w287) -> ()
      }
      event "timer set": Value Change {
        n245 = event-data() -> ()  [unwired: 1 in, 6 out]
        n246 = To Double Precision Float(number="Timer (ms)") -> (double precision float=w292:dbl)
        n247 = local read "FPenAcon"() -> (w295:refnum<vi>[])
        n248 = expression code="x/1000"(w292) -> (w291:dbl)
        n249 = call "SubVI Set Front panel elements.vi"("Enable elements (T)"=FALSE, "Array"=w295) -> ("error out"=w289:errorcluster)  [unwired: 9 in]
        n250 = local read "VISA"() -> (w290:refnum<visa-resource-name>)
        n251 = call "Configure Timer.vi"("error in (no error)"=w289, "Internal timer (2 s)"=w291, "VISA resource name"=w290) -> ("error out"=w288:errorcluster)  [unwired: 7 in, 1 out]
        n252 = local read "FPenAcon"() -> (w296:refnum<vi>[])
        n253 = call "SubVI Set Front panel elements.vi"("error in (passthrough)"=w288, "Array"=w296) -> ("error out"=w297:errorcluster)  [unwired: 9 in]
        n254 = local write "error"(w297) -> ()
      }
      event "timer get": Value Change {
        n255 = event-data() -> ()  [unwired: 1 in, 6 out]
        n256 = local read "FPenAcon"() -> (w304:refnum<vi>[])
        n257 = call "SubVI Set Front panel elements.vi"("Enable elements (T)"=FALSE, "Array"=w304) -> ("error out"=w302:errorcluster)  [unwired: 9 in]
        n258 = local read "VISA"() -> (w300:refnum<visa-resource-name>)
        n259 = call "Get Timer.vi"("error in (no error)"=w302, "VISA resource name"=w300) -> ("error out"=w301:errorcluster, "Internal Timer value (s)"=w299:dbl)  [unwired: 7 in, 1 out]
        n260 = local read "FPenAcon"() -> (w305:refnum<vi>[])
        n261 = expression code="int(x*1000)"(w299) -> (w298:dbl)
        n262 = call "SubVI Set Front panel elements.vi"("error in (passthrough)"=w301, "Array"=w305) -> ("error out"=w306:errorcluster)  [unwired: 9 in]
        n263 = local write "Timer (ms)"(w298) -> ()
        n264 = local write "error"(w306) -> ()
      }
      event "delay set": Value Change {
        n265 = event-data() -> ()  [unwired: 1 in, 6 out]
        n266 = local read "FPenAcon"() -> (w313:refnum<vi>[])
        n267 = expression code="x/1000"("Enable\nDelay (ms)") -> (w308:dbl)
        n268 = call "SubVI Set Front panel elements.vi"("Enable elements (T)"=FALSE, "Array"=w313) -> ("error out"=w310:errorcluster)  [unwired: 9 in]
        n269 = local read "VISA"() -> (w311:refnum<visa-resource-name>)
        n270 = call "Configure Delay.vi"("error in (no error)"=w310, "Delay (s)"=w308, "VISA resource name"=w311) -> ("error out"=w309:errorcluster)  [unwired: 7 in, 1 out]
        n271 = local read "FPenAcon"() -> (w314:refnum<vi>[])
        n272 = call "SubVI Set Front panel elements.vi"("error in (passthrough)"=w309, "Array"=w314) -> ("error out"=w315:errorcluster)  [unwired: 9 in]
        n273 = local write "error"(w315) -> ()
      }
      event "delay get": Value Change {
        n274 = event-data() -> ()  [unwired: 1 in, 6 out]
        n275 = local read "FPenAcon"() -> (w322:refnum<vi>[])
        n276 = call "SubVI Set Front panel elements.vi"("Enable elements (T)"=FALSE, "Array"=w322) -> ("error out"=w320:errorcluster)  [unwired: 9 in]
        n277 = local read "VISA"() -> (w318:refnum<visa-resource-name>)
        n278 = call "Get Delay.vi"("error in (no error)"=w320, "VISA resource name"=w318) -> ("error out"=w319:errorcluster, "Delay (s)"=w317:dbl)  [unwired: 7 in, 1 out]
        n279 = local read "FPenAcon"() -> (w323:refnum<vi>[])
        n280 = expression code="int(x*1000)"(w317) -> (w316:dbl)
        n281 = call "SubVI Set Front panel elements.vi"("error in (passthrough)"=w319, "Array"=w323) -> ("error out"=w324:errorcluster)  [unwired: 9 in]
        n282 = local write "Enable\nDelay (ms)"(w316) -> ()
        n283 = local write "error"(w324) -> ()
      }
      event "check channels", "dummy for event \"check channels\"": Value Change {
        # "this is only to get possibility\nto start this event case\neven if button \"check channels\"\nis latching"
        n284 = event-data() -> ()  [unwired: 1 in, 6 out]
        n285 = local read "FPenAcon"() -> (w339:refnum<vi>[])
        n286 = call "SubVI Set Front panel elements.vi"("Enable elements (T)"=FALSE, "Array"=w339) -> ("error out"=w332:errorcluster)  [unwired: 9 in]
        n287 = local read "VISA"() -> (w333:refnum<visa-resource-name>)
        n288 = local read "Guards ref array"() -> (w329:refnum<vi>[][])
        n289 = local read "Slaves ref array"() -> (w335:refnum<vi>[][])
        n290 = call "Get Slaves Number & Positions.vi"("error in (no error)"=w332, "VISA resource name"=w333) -> ("error out"=w330:errorcluster, "Connected Slaves"=w334:bool[], "No. of Slaves"=w336:u32)  [unwired: 6 in, 1 out]
        "Connected\nboards" <- w334
        n291 = local write "No. of connected slave boards:"(w336) -> ()
        n292 = for {
          tunnel: w335 -> [w347] mode=indexing
          tunnel: w334 -> [w343] mode=indexing
          shift-right: [w344] -> w331
          shift-left: w330 -> [w346]
          tunnel: w329 -> [w342] mode=indexing
          n293 = call "SubVI Set Front panel elements.vi"("Enable elements (T)"=w343, "error in (passthrough)"=w346, "Array"=w347) -> ("error out"=w345:errorcluster)  [unwired: 8 in]
          n294 = call "SubVI Set Front panel elements.vi"("Enable elements (T)"=w343, "error in (passthrough)"=w345, "Array"=w342) -> ("error out"=w344:errorcluster)  [unwired: 8 in]
        }
        n295 = for {
          N: 2 -> [_]
          shift-right: [w351] -> w326
          shift-left: w331 -> [w350]
          i -> [w349]
          n296 = Increment(x=w349) -> (x+1=w348:i32)
          n297 = for {
            N: 6 -> [_]
            shift-right: [w360] -> w351
            shift-left: w350 -> [w359]
            tunnel: w348 -> [w354]
            i -> [w357]
            # "#XXX no way how to check guard status?"
            n298 = local read "VISA"() -> (w358:refnum<visa-resource-name>)
            n299 = Increment(x=w357) -> (x+1=w355:i32)
            n300 = call "Get Channel Status.vi"("Channel"=w354, "Slave"=w355, "error in (no error)"=w359, "VISA resource name"=w358) -> ("error out"=w360:errorcluster, "Channel Enabled"=w353:bool)  [unwired: 5 in, 1 out]
            n301 = local read "Slaves ref array"() -> (w356:refnum<vi>[][])
            n302 = call "SubVI Set FP Channel-Guard value.vi"("Value"=w353, "Ch ID"=w354, "Slave ID"=w355, "Slaves ref array"=w356) -> ()  [unwired: 7 in, 1 out]
          }
        }
        n303 = Enqueue Element(queue=w327, element="slaves update", error in (no error)=w326) -> (error out=w325:errorcluster)  [unwired: 1 in, 2 out]
        n304 = local read "FPenAcon"() -> (w340:refnum<vi>[])
        n305 = call "SubVI Set Front panel elements.vi"("error in (passthrough)"=w325, "Array"=w340) -> ("error out"=w341:errorcluster)  [unwired: 9 in]
        n306 = local write "error"(w341) -> ()
      }
      event "Get Status": Value Change {
        n307 = event-data() -> ()  [unwired: 1 in, 6 out]
        n308 = local read "FPenAcon"() -> (w379:refnum<vi>[])
        n309 = call "SubVI Set Front panel elements.vi"("Enable elements (T)"=FALSE, "Array"=w379) -> ("error out"=w374:errorcluster)  [unwired: 9 in]
        n310 = local read "VISA"() -> (w375:refnum<visa-resource-name>)
        n311 = call "Get MX Status.vi"("error in (no error)"=w374, "VISA resource name"=w375) -> ("error out"=w373:errorcluster, "Ready?"=→"Ready?":bool, "Enabled"=→"Enabled":bool, "TRG Polarity Positive"=w368:bool, "Local?"=w372:bool, "TRG External"=w364:bool)  [unwired: 3 in, 1 out]
        n312 = local read "FPenAcon"() -> (w380:refnum<vi>[])
        n313 = Select(t=enum32{"Remote", "Local"}."Local" ("Operation"), s=w372, f=enum32{"Remote", "Local"}."Remote" ("Operation")) -> (s? t:f=w369:enum32{"Remote", "Local"})
        n314 = Select(t=enum32{"Positive", "Negative"}."Positive" ("Trigger polarity"), s=w368, f=enum32{"Positive", "Negative"}."Negative" ("Trigger polarity")) -> (s? t:f=w365:enum32{"Positive", "Negative"})
        n315 = Select(t=enum32{"Internal", "External"}."External" ("Trigger source"), s=w364, f=enum32{"Internal", "External"}."Internal" ("Trigger source")) -> (s? t:f=w361:enum32{"Internal", "External"})
        n316 = call "SubVI Set Front panel elements.vi"("error in (passthrough)"=w373, "Array"=w380) -> ("error out"=w381:errorcluster)  [unwired: 9 in]
        n317 = local write "Operation"(w369) -> ()
        n318 = local write "Trigger polarity"(w365) -> ()
        n319 = local write "Trigger source"(w361) -> ()
        n320 = local write "error"(w381) -> ()
      }
      event "no sequences get": Value Change {
        n321 = event-data() -> ()  [unwired: 1 in, 6 out]
        n322 = local read "FPenAcon"() -> (w387:refnum<vi>[])
        n323 = call "SubVI Set Front panel elements.vi"("Enable elements (T)"=FALSE, "Array"=w387) -> ("error out"=w385:errorcluster)  [unwired: 9 in]
        n324 = local read "VISA"() -> (w383:refnum<visa-resource-name>)
        n325 = call "Get Number of Sequences.vi"("error in (no error)"=w385, "VISA resource name"=w383) -> ("error out"=w384:errorcluster, "Number of sequences"=w382:i32)  [unwired: 7 in, 1 out]
        n326 = local read "FPenAcon"() -> (w388:refnum<vi>[])
        n327 = local write "Number of sequence lines:"(w382) -> ()
        n328 = call "SubVI Set Front panel elements.vi"("error in (passthrough)"=w384, "Array"=w388) -> ("error out"=w389:errorcluster)  [unwired: 9 in]
        n329 = local write "error"(w389) -> ()
      }
      event "sequence editor": Value Change {
        n330 = event-data() -> ()  [unwired: 1 in, 6 out]
        n331 = Enqueue Element(queue=w391, element="FP open") -> ()  [unwired: 2 in, 3 out]
      }
      event "Load sq to MX": Value Change {
        n332 = event-data() -> ()  [unwired: 1 in, 6 out]
        n333 = disable-structure shown="Default" {
          disable-tunnel: w396 -> [w428]
          disable-tunnel: [w413] -> w395
          disable-tunnel: [w412] -> w394
          frame Enabled {
            # "Get actual values from Sequence editor.vi"
            n334 = property class="VI"(reference=w428) -> ("Panel"=w427:refnum<vi>)  [unwired: 1 in, 2 out]
            n335 = property class="Pnl"(reference=w427) -> (reference out=w414:refnum<vi>, "Controls[]"=w415:refnum<vi>[])  [unwired: 1 in, 1 out]
            n336 = Close Reference(reference=w414) -> ()  [unwired: 1 in, 1 out]
            n337 = Close Reference(reference=w415) -> ()  [unwired: 1 in, 1 out]
            n338 = for {
              tunnel: w415 -> [w430] mode=indexing
              tunnel: [w429] -> w417 mode=indexing
              n339 = property class="Ctl"(reference=w430) -> ("Label.Text"=w429:string)  [unwired: 1 in, 2 out]
            }
            n340 = call "Search Unsorted 1D Array.vim"("element"="Sequence" ("Label.Text"), "unsorted 1D array"=w417) -> ("index of element"=w419:i32)  [unwired: 9 in]
            n341 = call "Search Unsorted 1D Array.vim"("element"="Timing\ndelay" ("Label.Text"), "unsorted 1D array"=w417) -> ("index of element"=w425:i32)  [unwired: 9 in]
            n342 = Index Array(array=w415, index=w419) -> (element=w420:refnum<vi>)
            n343 = property class="Ctl"(reference=w420) -> ("Value"=w421:variant)  [unwired: 1 in, 2 out]
            n344 = Index Array(array=w415, index=w425) -> (element=w424:refnum<vi>)
            n345 = property class="Ctl"(reference=w424) -> ("Value"=w423:variant)  [unwired: 1 in, 2 out]
            n346 = Variant To Data(type=u8[] [] ("Ch. bytes 2"), Variant=w423) -> (data=w412:u8[])  [unwired: 1 in, 1 out]
            n347 = Variant To Data(type=bool[][] [], Variant=w421) -> (data=w413:bool[][])  [unwired: 1 in, 1 out]
          }
        }
        n348 = Array Size(array=w394) -> (size(s)=w393:i32)
        n349 = Equal To 0?(x=w393) -> (x = 0?=w392:bool)
        n350 = case shown="False" w392 {
          tunnel: w395 -> [w402 _]
          tunnel: w394 -> [w401 _]
          frame False {
            n351 = local read "FPenAcon"() -> (w406:refnum<vi>[])
            n352 = call "Sequences to Bytes.vi"("Channel states"=w402) -> ("Ch. bytes 2"=w409:u8[], "Ch. bytes 1"=w410:u8[])  [unwired: 9 in]
            n353 = call "SubVI Set Front panel elements.vi"("Enable elements (T)"=FALSE, "Array"=w406) -> ("error out"=w404:errorcluster)  [unwired: 9 in]
            n354 = local read "VISA"() -> (w403:refnum<visa-resource-name>)
            n355 = call "Load Sequences.vi"("Byte 2 Ch."=w409, "Byte 3 Timing Delay"=w401, "Byte 1 Ch."=w410, "error in (no error)"=w404, "VISA resource name"=w403) -> ("error out"=w399:errorcluster, "VISA resource name out"=w397:refnum<visa-resource-name>)  [unwired: 5 in]
            n356 = local read "FPenAcon"() -> (w407:refnum<vi>[])
            n357 = call "Get Number of Sequences.vi"("error in (no error)"=w399, "VISA resource name"=w397) -> ("error out"=w398:errorcluster, "Number of sequences"=w400:i32)  [unwired: 7 in, 1 out]
            n358 = call "SubVI Set Front panel elements.vi"("error in (passthrough)"=w398, "Array"=w407) -> ("error out"=w408:errorcluster)  [unwired: 9 in]
            n359 = local write "error"(w408) -> ()
            n360 = local write "Number of sequence lines:"(w400) -> ()
          }
          frame True {
            n361 = One Button Dialog(message="Sequence matrix is empty.\nUse sequence editor to create\nsequence or load sequence\nfrom file.") -> ()  [unwired: 1 in, 1 out]
          }
        }
      }
      event "set sq line": Value Change {
        n362 = event-data() -> ()  [unwired: 1 in, 6 out]
        n363 = disable-structure shown="Default" {
          disable-tunnel: w444 -> [w455]
          disable-tunnel: [w445] -> w439
          frame Enabled {
            # "Get actual values from Sequence editor.vi"
            n364 = property class="VI"(reference=w455) -> ("Panel"=w454:refnum<vi>)  [unwired: 1 in, 2 out]
            n365 = property class="Pnl"(reference=w454) -> (reference out=w446:refnum<vi>, "Controls[]"=w447:refnum<vi>[])  [unwired: 1 in, 1 out]
            n366 = Close Reference(reference=w446) -> ()  [unwired: 1 in, 1 out]
            n367 = Close Reference(reference=w447) -> ()  [unwired: 1 in, 1 out]
            n368 = for {
              tunnel: w447 -> [w457] mode=indexing
              tunnel: [w456] -> w449 mode=indexing
              n369 = property class="Ctl"(reference=w457) -> ("Label.Text"=w456:string)  [unwired: 1 in, 2 out]
            }
            n370 = call "Search Unsorted 1D Array.vim"("element"="Sequence" ("Label.Text"), "unsorted 1D array"=w449) -> ("index of element"=w451:i32)  [unwired: 9 in]
            n371 = Index Array(array=w447, index=w451) -> (element=w452:refnum<vi>)
            n372 = property class="Ctl"(reference=w452) -> ("Value"=w453:variant)  [unwired: 1 in, 2 out]
            n373 = Variant To Data(type=bool[][] [], Variant=w453) -> (data=w445:bool[][])  [unwired: 1 in, 1 out]
          }
        }
        n374 = local read "FPenAcon"() -> (w442:refnum<vi>[])
        n375 = Decrement(x="Set to sequence line:") -> (x-1=w431:i32)
        n376 = Index Array(array=w439, index (row)=w431) -> (element=w438:bool[])  [unwired: 1 in]
        n377 = call "SubVI Set Front panel elements.vi"("Enable elements (T)"=FALSE, "Array"=w442) -> ("error out"=w440:errorcluster)  [unwired: 9 in]
        n378 = local read "VISA"() -> (w437:refnum<visa-resource-name>)
        n379 = call "Set Sequence Line.vi"("error in (no error)"=w440, "Sequence Line"=w438, "VISA resource name"=w437) -> ("error out"=w436:errorcluster)  [unwired: 7 in, 1 out]
        n380 = local read "FPenAcon"() -> (w443:refnum<vi>[])
        n381 = call "SubVI Set Front panel elements.vi"("error in (passthrough)"=w436, "Array"=w443) -> ("error out"=w435:errorcluster)  [unwired: 9 in]
        n382 = property on="dummy for event \"check channels\"" class="Bool (strict)"(error in=w435, "Val(Sgnl)"=TRUE) -> (error out=w434:errorcluster)  [unwired: 1 in, 1 out]
        n383 = local write "error"(w434) -> ()
      }
      event "Get sq from MX": Value Change {
        n384 = event-data() -> ()  [unwired: 1 in, 6 out]
        n385 = local read "FPenAcon"() -> (w459:refnum<vi>[])
        n386 = call "SubVI Set Front panel elements.vi"("Enable elements (T)"=FALSE, "Array"=w459) -> ("error out"=w477:errorcluster)  [unwired: 9 in]
        n387 = local read "VISA"() -> (w475:refnum<visa-resource-name>)
        n388 = call "Get Sequences.vi"("error in (no error)"=w477, "VISA resource name"=w475) -> ("error out"=w476:errorcluster, "Byte 3 Delay"=w469:u8[], "Byte 2 Ch."=w472:u8[], "Byte 1 Ch."=w473:u8[])  [unwired: 5 in, 1 out]
        n389 = local read "FPenAcon"() -> (w478:refnum<vi>[])
        n390 = Array Size(array=w469) -> (size(s)=w474:i32)
        n391 = call "Bytes to Sequences.vi"("Ch. bytes 2"=w472, "Ch. bytes 1"=w473) -> ("Array"=w470:bool[][])  [unwired: 9 in]
        n392 = call "SubVI Set Front panel elements.vi"("error in (passthrough)"=w476, "Array"=w478) -> ("error out"=w479:errorcluster)  [unwired: 9 in]
        n393 = local write "Number of sequence lines:"(w474) -> ()
        n394 = local write "error"(w479) -> ()
        n395 = disable-structure shown="Default" {
          disable-tunnel: w471 -> [w493]
          disable-tunnel: w470 -> [w482]
          disable-tunnel: w469 -> [w481]
          disable-tunnel: w468 -> [w480]
          disable-tunnel: [w480] -> w460
          frame Enabled {
            # "Push actual values to Sequence editor.vi"
            n396 = property class="VI"(reference=w493) -> ("Panel"=w492:refnum<vi>)  [unwired: 1 in, 2 out]
            n397 = property class="Pnl"(reference=w492) -> (reference out=w483:refnum<vi>, "Controls[]"=w484:refnum<vi>[])  [unwired: 1 in, 1 out]
            n398 = Close Reference(reference=w483) -> ()  [unwired: 1 in, 1 out]
            n399 = Close Reference(reference=w484) -> ()  [unwired: 1 in, 1 out]
            n400 = for {
              tunnel: w484 -> [w495] mode=indexing
              tunnel: [w494] -> w485 mode=indexing
              n401 = property class="Ctl"(reference=w495) -> ("Label.Text"=w494:string)  [unwired: 1 in, 2 out]
            }
            n402 = call "Search Unsorted 1D Array.vim"("element"="Sequence" ("Label.Text"), "unsorted 1D array"=w485) -> ("index of element"=w487:i32)  [unwired: 9 in]
            n403 = call "Search Unsorted 1D Array.vim"("element"="Timing\ndelay" ("Label.Text"), "unsorted 1D array"=w485) -> ("index of element"=w490:i32)  [unwired: 9 in]
            n404 = Index Array(array=w484, index=w487) -> (element=w488:refnum<vi>)
            n405 = property class="Ctl"(reference=w488, "Value"=w482) -> ()  [unwired: 1 in, 2 out]
            n406 = Index Array(array=w484, index=w490) -> (element=w489:refnum<vi>)
            n407 = property class="Ctl"(reference=w489, "Value"=w481) -> ()  [unwired: 1 in, 2 out]
          }
        }
        n408 = Enqueue Element(queue=w460, element="sequence fill missing collumns") -> (queue out=w464:refnum<queue>, error out=w467:errorcluster)  [unwired: 2 in, 1 out]
        n409 = Enqueue Element(queue=w464, element="index timing update", error in (no error)=w467) -> (queue out=w465:refnum<queue>, error out=w466:errorcluster)  [unwired: 1 in, 1 out]
        n410 = Enqueue Element(queue=w465, element="scrollbar sync", error in (no error)=w466) -> ()  [unwired: 1 in, 3 out]
      }
    }
  }
  n411 = flat-sequence {
    tunnel: w10 -> [w499]
    tunnel: w11 -> [w496]
    tunnel: w14 -> [_]
    tunnel: [w499] -> w5
    tunnel: [w497] -> w3
    tunnel: [w506] -> w7
    tunnel: ["Do full quit? (T)"] -> w6
    tunnel: w5 -> [w506]
    tunnel: [w500] -> w4
    tunnel: w3 -> [w500]
    tunnel: w6 -> [w511]
    tunnel: w7 -> [w510]
    tunnel: w4 -> [w508]
    frame #0 {
      n412 = Enqueue Element(queue=w496, element="quit") -> (error out=w497:errorcluster)  [unwired: 2 in, 2 out]
    }
    frame #1 {
      n413 = property class="VI"() -> ("FP.State"=w505:T2)  [unwired: 2 in, 2 out]
      n414 = Not Equal?(x=w505, y=T2."Closed") -> (x != y?=w502:bool)
      n415 = Compound Arithmetic op=AND(invert "Do full quit? (T)", w502) -> (w501:bool)
      n416 = case shown="True" w501 {
        tunnel: w506 -> [_ w507]
        frame False {
        }
        frame True {
          n417 = invoke class="VI" method="FP.Close"(reference=w507) -> ()  [unwired: 2 in, 3 out]
        }
      }
    }
    frame #2 {
      n418 = local read "VISA"() -> (w514:refnum<visa-resource-name>)
      n419 = call "Close.vi"("VISA resource name"=w514) -> ("error out"=w513:errorcluster)  [unwired: 10 in]
      n420 = Close Reference(reference=w510) -> (error out=w509:errorcluster)  [unwired: 1 in]
      n421 = Merge Errors(w513, w508, w509) -> (w512:errorcluster)
      "error" <- w512
      n422 = case shown="True" w511 {
        tunnel: w512 -> [_ w515]
        frame False {
        }
        frame True {
          n423 = disable-structure shown="RUN_TIME_ENGINE==True" {
            disable-tunnel: w515 -> [_ _]
            frame condition #0 (active) {
              n424 = Stop(stop? (T)=TRUE) -> ()
            }
            frame condition #1 {
              n425 = Quit LabVIEW(quit? (T)=TRUE) -> ()
            }
          }
        }
      }
    }
  }
